vi "Main_02B.vi"() -> ()   [LabVIEW 2025]
uses:
  <vilib>/Utility/error.llb/Trim Whitespace One-Sided.vi
  Utility/Universal Utility/TypeDefs_Utility/Cluster_Row-Column.ctl
  9e3f57c0-2ef8-4495-8287-c6a42a5fb955.vi
  Utility/Universal Utility/TypeDefs_Utility/ENUM_4 Directions U-D-L-R.ctl
  Utility/Universal Utility/TypeDefs_Utility/ENUM_8 Directions U-D-L-R.ctl
panel:
  out "string array":string[](array[string])
  out "U64 -1":u64
  out "Invalid Array":u64[](array[numeric])
  out "MATCH":bool
  in  "Select Data":enum32{"Example", "Puzzle"}(tab)
  in  "EX Target":u64=4174379265
  in  "Example":string="11-22,95-115,998-1012,1188511880-1188511890,222220-222224,\n1698522-1698528,446443-446449,38593856-38593862,565653-565659,\n824824821-824824827,2121212118-2121212124"
  in  "Puzzle":string="874324-1096487,6106748-6273465,1751-4283,294380-348021,5217788-5252660,828815656-828846474,66486-157652,477-1035,20185-55252,17-47,375278481-375470130,141-453,33680490-33821359,88845663-88931344,621298-752726,21764551-21780350,58537958-58673847,9983248-10042949,4457-9048,9292891448-9292952618,4382577-4494092,199525-259728,9934981035-9935011120,6738255458-6738272752,8275916-8338174,1-15,68-128,7366340343-7366538971,82803431-82838224,72410788-72501583"
  in  "Puzzle Target":u64=54486209192
  out "Answer":u64
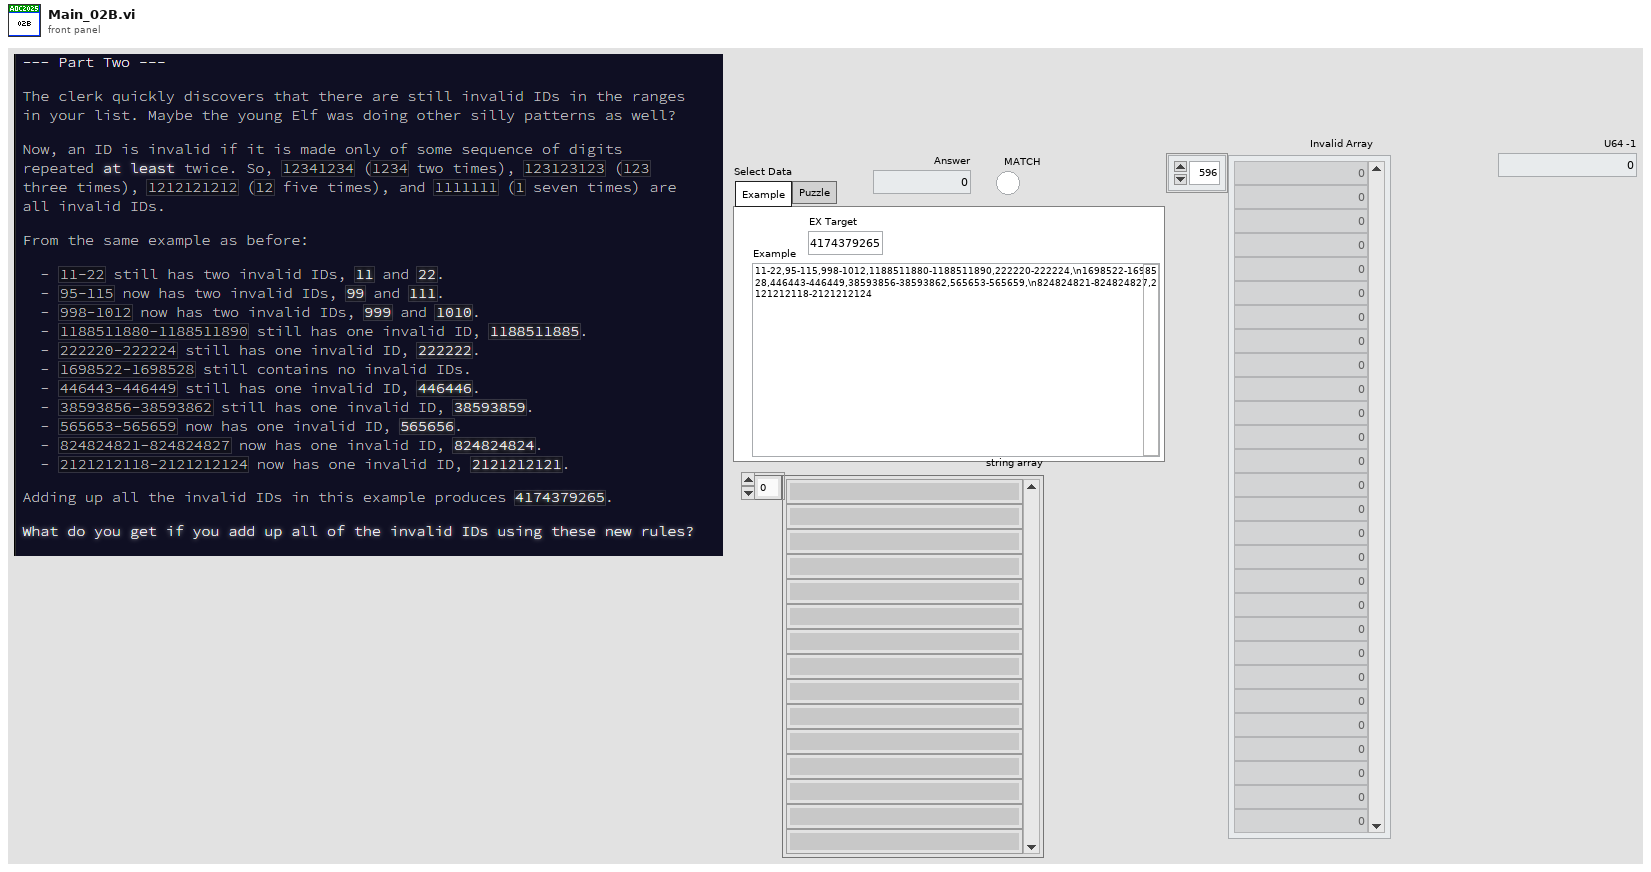
[diagram p1: front panel]
types:
  T1 = typedef "ENUM_8 Directions U-D-L-R.ctl" = enum16{"Up;-1,0", "Up-Right;-1,1", "Right;0,1", "Down-Right;1,1", "Down;1,0", "Down-Left;1,-1", "Left;0,-1", "Up-Left;-1,-1"}
  T2 = typedef "ENUM_4 Directions U-D-L-R.ctl" = enum16{"Up;-1,0", "Right;0,1", "Down;1,0", "Left;0,-1"}
  T3 = typedef "Cluster_Row-Column.ctl" = cluster{"R":i32, "C":i32}
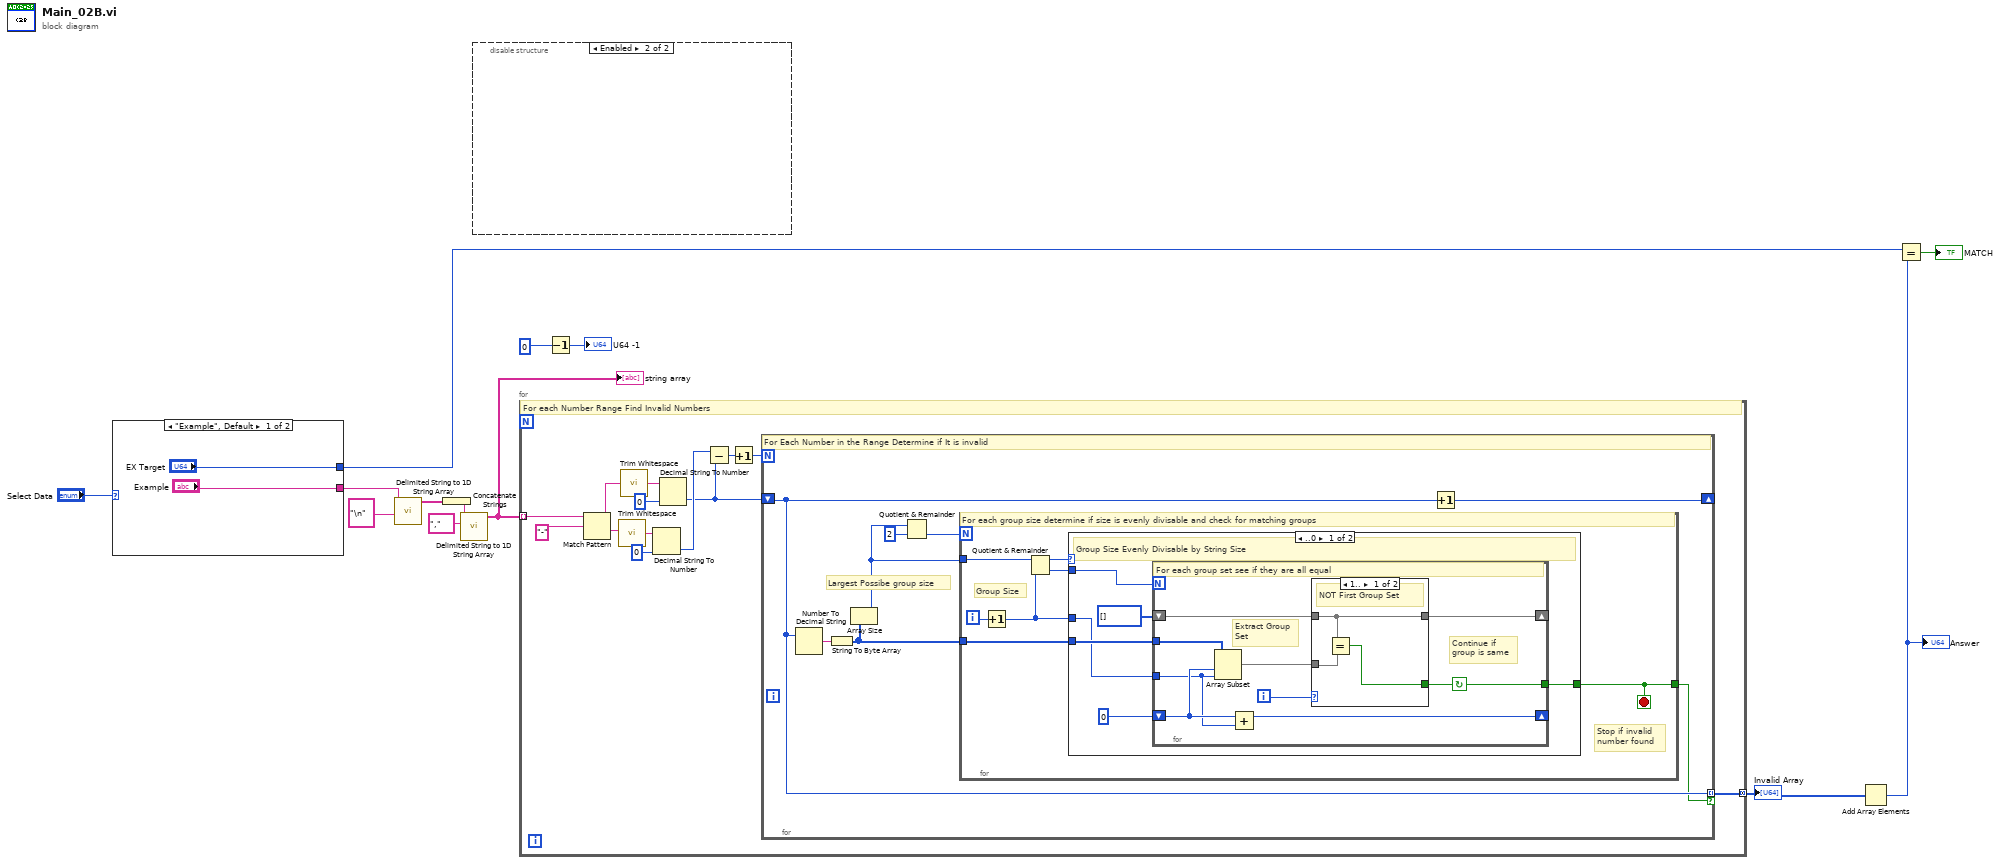
[diagram p0: block diagram]
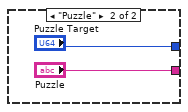
[diagram p2: hidden frame]
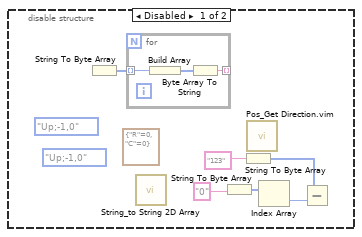
[diagram p3: hidden frame]
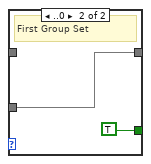
[diagram p4: hidden frame]
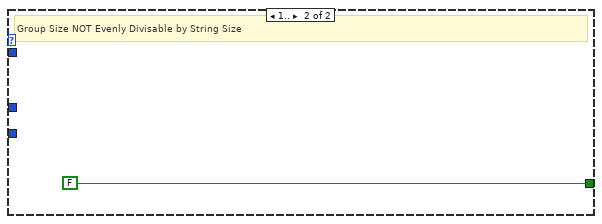
[diagram p5: hidden frame]
diagram:
  n1 = case shown="\"Example\", Default" "Select Data" {
    tunnel: ["Example" "Puzzle"] -> w5
    tunnel: ["EX Target" "Puzzle Target"] -> w10
    frame "Example", Default {
    }
    frame "Puzzle" {
    }
  }
  n2 = call <vilib>:"Delimited String to 1D String Array.vi"("delimiter"="\n" ("delimiter (Tab)"), "delimited string"=w5) -> ("string array"=w3:string[])  [unwired: 9 in]
  n3 = Concatenate Strings(w3) -> (w2:string)
  n4 = call <vilib>:"Delimited String to 1D String Array.vi"("delimiter"="," ("delimiter (Tab)"), "delimited string"=w2) -> ("string array"=w13:string[])  [unwired: 9 in]
  "string array" <- w13
  n5 = disable-structure shown="Enabled" {
    frame Disabled {
      (unwired) ENUM_8_Directions_U-D-L-R."Up;-1,0" ("Direction 8")
      (unwired) ENUM_4_Directions_U-D-L-R."Up;-1,0" ("Direction")
      (unwired) T3 {"R"=0, "C"=0} ("Position")
      n6 = String To Byte Array() -> (unsigned byte array=w18:u8[])  [unwired: 1 in]
      n7 = for {
        tunnel: w18 -> [w26] mode=indexing
        tunnel: [w24] -> _ mode=indexing
        n8 = Build Array(w26) -> (w25:u8[])
        n9 = Byte Array To String(unsigned byte array=w25) -> (string=w24:string)
      }
      n10 = call "String_to String 2D Array.vi"() -> ()  [unwired: 11 in, 1 out]
      n11 = String To Byte Array(string="0") -> (unsigned byte array=w21:u8[])
      n12 = String To Byte Array(string="123") -> (unsigned byte array=w19:u8[])
      n13 = call "Pos_Get Direction.vim"() -> ()  [unwired: 11 in, 1 out]
      n14 = Index Array(array=w21) -> (element=w20:u8)  [unwired: 1 in]
      n15 = Subtract(x=w19, y=w20) -> ()  [unwired: 1 out]
    }
    frame Enabled {
    }
  }
  n16 = for {
    tunnel: w13 -> [w39] mode=indexing
    tunnel: [w27] -> w9 mode=concatenating
    # "For each Number Range Find Invalid Numbers"
    n17 = Match Pattern(string=w39, regular expression="-" ("delimiter")) -> (before substring=w37:string, after substring=w35:string)  [unwired: 1 in, 2 out]
    n18 = call <vilib>:"Trim Whitespace.vi"("string"=w35) -> ("trimmed string"=w34:string)  [unwired: 1 in]
    n19 = call <vilib>:"Trim Whitespace.vi"("string"=w37) -> ("trimmed string"=w36:string)  [unwired: 1 in]
    n20 = Decimal String To Number(string=w34, default (0L)=u64 0 ("default (0 I32)")) -> (number=w31:u64)  [unwired: 1 in, 1 out]
    n21 = Decimal String To Number(string=w36, default (0L)=u64 0 ("default (0 I32)")) -> (number=w28:u64)  [unwired: 1 in, 1 out]
    n22 = Subtract(x=w31, y=w28) -> (x-y=w30:u64)
    n23 = Increment(x=w30) -> (x+1=w29:u64)
    n24 = for {
      N: w29 -> [_]
      shift-right: [w47] -> _
      shift-left: w28 -> [w45]
      tunnel: [w45] -> w27 mode=indexing if=w42
      # "Largest Possibe group size"
      # "For Each Number in the Range Determine if It is invalid"
      n25 = Number To Decimal String(number=w45) -> (decimal integer string=w44:string)  [unwired: 1 in]
      n26 = String To Byte Array(string=w44) -> (unsigned byte array=w43:u8[])
      n27 = Array Size(array=w43) -> (size(s)=w40:i32)
      n28 = Quotient & Remainder(x=w40, y=2) -> (floor(x/y)=w41:i32)  [unwired: 1 out]
      n29 = for {
        N: w41 -> [_]
        tunnel: w43 -> [w54]
        tunnel: [w48] -> w42
        tunnel: w40 -> [w52]
        i -> [w53]
        stop <- w48 stop-if-true
        # "Group Size"
        # "Stop if invalid\nnumber found"
        # "For each group size determine if size is evenly divisable and check for matching groups"
        n30 = Increment(x=w53) -> (x+1=w49:i32)
        n31 = Quotient & Remainder(x=w52, y=w49) -> (x-y*floor(x/y)=w51:i32, floor(x/y)=w50:i32)
        n32 = case shown="..0" w51 {
          tunnel: w54 -> [w59 _]
          tunnel: [w55 FALSE] -> w48
          tunnel: w50 -> [w60 _]
          tunnel: w49 -> [w57 _]
          frame ..0 {
            # "Group Size Evenly Divisable by String Size"
            n33 = for {
              N: w60 -> [_]
              tunnel: w59 -> [w68]
              shift-right: [w64] -> _
              shift-left: u8[] [] -> [w62]
              shift-right: [w65] -> _
              shift-left: 0 -> [w67]
              tunnel: w57 -> [w66]
              tunnel: [w61] -> w55
              i -> [w69]
              stop <- w61 continue-if-true
              # "Continue if\ngroup is same"
              # "Extract Group\nSet"
              # "For each group set see if they are all equal"
              n34 = Array Subset(array=w68, index=w67, length=w66) -> (w63:u8[])
              n35 = Add(x=w67, y=w66) -> (x+y=w65:i32)
              n36 = case shown="1.." w69 {
                tunnel: [w70 w74] -> w64
                tunnel: w63 -> [w72 w74]
                tunnel: w62 -> [w70 _]
                tunnel: [w71 TRUE] -> w61
                frame 1.. {
                  # "NOT First Group Set"
                  n37 = Equal?(x=w70, y=w72) -> (x = y?=w71:bool)
                }
                frame ..0 {
                  # "First Group Set"
                }
              }
            }
          }
          frame 1.. {
            # "Group Size NOT Evenly Divisable by String Size"
          }
        }
      }
      n38 = Increment(x=w45) -> (x+1=w47:u64)
    }
  }
  "Invalid Array" <- w9
  n39 = Decrement(x=u64 0 ("sum")) -> (x-1=→"U64 -1":u64)
  n40 = Add Array Elements(numeric array=w9) -> (sum=w8:u64)
  "Answer" <- w8
  n41 = Equal?(x=w10, y=w8) -> (x = y?=→"MATCH":bool)
